vi "From JSON.vi"(8 "error in (no error)":errorcluster, 10 "JSON":string, 11 "Double Float in":refnum<class "Abs_Complex Double Float.lvclass">) -> (0 "error out":errorcluster, 3 "Double Float out":refnum<class "Abs_Complex Double Float.lvclass">)   [LabVIEW 2021, in "Abs_Complex Double Float.lvclass"]
uses:
  Abs_Complex Double Float.lvclass
  C:/Program Files (x86)/National Instruments/LabVIEW 2021/vi.lib/TSA/Abstract Data Classes/Abs_Types/Type/Abs_Type.lvclass
  Support/Type.ctl
  433cb2d8-b6c1-4669-8d2e-08263996b4f8.vi
  <vilib>/JDP Science/JSONtext/Find Item.vi
  <vilib>/JDP Science/JSONtext/Next JSON Value.vi
  <vilib>/JDP Science/JSONtext/String Subset.vi
  <vilib>/JDP Science/JSONtext/Parsing/Advance past next JSON Value (inlined COPY).vi
  <vilib>/JDP Science/JSONtext/Parsing/Advance past whitespace.vi
  <vilib>/JDP Science/JSONtext/Parsing/Advance past String.vi
  <vilib>/JDP Science/JSONtext/Parsing/Advance past Number.vi
  <vilib>/JDP Science/JSONtext/Parsing/Advance past Line Ending.vi
  <vilib>/Utility/LVClass/Get LV Class Name.vi
  <vilib>/JDP Science/JSONtext/Parsing/Parse Full Path or Item Name.vi
  <vilib>/JDP Science/JSONtext/Parsing/Advance past Array.vi
  <vilib>/JDP Science/JSONtext/Parsing/Advance past Object.vi
  <vilib>/JDP Science/JSONtext/support/Error Cluster From Code.vi
  <vilib>/JDP Science/JSONtext/Offset/Find Item Locations by Path.vi
  <vilib>/JDP Science/JSONtext/JSON text to Variant.vi
  <vilib>/JDP Science/JSONtext/LVClass Serializer/JSONtext LVClass Serializer.lvclass
  Floating Point/Abs_Floating Point.lvclass
  Type/Abs_Type.lvclass
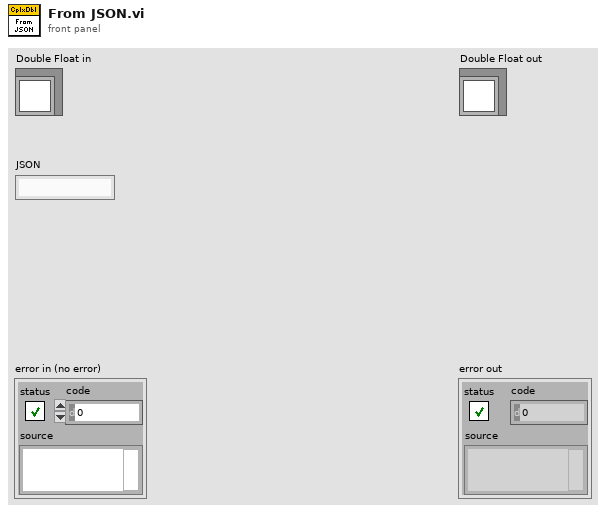
[diagram p1: front panel]
types:
  T1 = typedef "Abs_Complex Double Float.lvclass/Type.ctl" = cdb
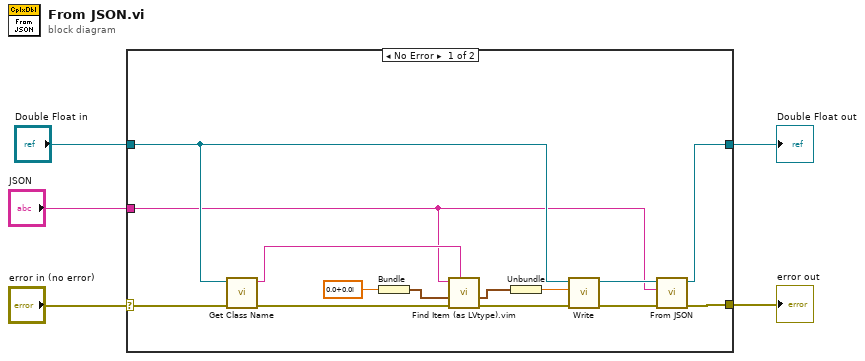
[diagram p0: block diagram]
diagram:
  n1 = case shown="No Error" "error in (no error)" {
    selector: "error in (no error)" -> [w15 w20]
    tunnel: [w19 w20] -> w2
    tunnel: [w18 w21] -> w1
    tunnel: "JSON" -> [w6 _]
    tunnel: "Double Float in" -> [w8 w21]
    frame No Error {
      n2 = call "Get Class Name.vi"("error in (no error)"=w15, "Abs_Type in"=w8) -> ("error out"=w13:errorcluster, "class name"=w14:string)  [unwired: 8 in]
      n3 = Bundle("Value"=T1 0.0+0.0i) -> (w16:cluster{"Value":T1})  [unwired: 1 in]
      n4 = call "Find Item (as LVtype).vim"("$Path or Item Name"=w14, "error in (no error)"=w13, "Data Type and Default Value"=w16, "JSON"=w6) -> ("error out"=w12:errorcluster, "Data"=w17:cluster{"Value":T1})  [unwired: 4 in, 2 out]
      n5 = Unbundle(w17) -> ("Value"=w9:T1)
      n6 = call-dynamic "Write.vi"("error in (no error)"=w12, "Value"=w9, "Double Float.lvclass_340760 in"=w8) -> ("error out"=w11:errorcluster, "Double Float.lvclass_340760 out"=w10:refnum<class "Abs_Complex Double Float.lvclass">)  [unwired: 7 in]
      n7 = call-parent "From JSON.vi"("error in (no error)"=w11, "JSON"=w6, "Type in"=w10) -> ("error out"=w19:errorcluster, "Type out"=w18:refnum<class "Abs_Complex Double Float.lvclass">)  [unwired: 7 in]
    }
    frame Error {
    }
  }
  "error out" <- w2
  "Double Float out" <- w1
